vi "Cleanup.vi"(8 "error in (no error)":errorcluster, 11 "PanelArray in":refnum<class "PanelArray.lvclass">) -> (0 "error out":errorcluster)   [LabVIEW 2018, in "OOPanel.lvlib" / "PanelArray.lvclass"]
uses:
  PanelArray.lvclass
  PanelArray.lvclass/PanelArray.ctl
  Panel/Panel.lvclass
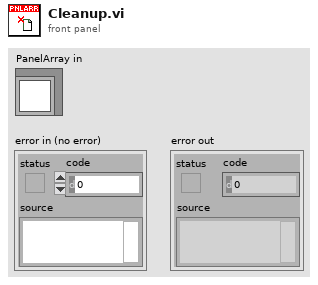
[diagram p1: front panel]
types:
  T1 = typedef "OOPanel.lvlib/PanelArray.lvclass/Ref Data.ctl" = cluster{"State":T2, "Refs":T3, "Events":T4, "Scrolling":T5, "Panels":T6}
  T2 = typedef "OOPanel.lvlib/PanelArray.lvclass/State.ctl" = cluster{"Defer Updates":bool, "Running":bool, "Dynamic Sizing":bool, "Borders":bool}
  T3 = typedef "OOPanel.lvlib/PanelArray.lvclass/Refs.ctl" = cluster{"SubPanels":refnum<vi>[], "Scrollbar":refnum<vi>, "Owning Panel":refnum<vi>}
  T4 = typedef "OOPanel.lvlib/PanelArray.lvclass/Events.ctl" = cluster{"Close":refnum<user-event>}
  T5 = typedef "OOPanel.lvlib/PanelArray.lvclass/Scrolling.ctl" = cluster{"Size":i32, "Max":i32, "Current":i32, "Top Index":i32, "Heights":i32[]}
  T6 = typedef "OOPanel.lvlib/PanelArray.lvclass/Panels.ctl" = cluster{"All":refnum<class "Panel.lvclass">[], "Visible":refnum<class "Panel.lvclass">[], "Blank":refnum<class "ArrayBlank.lvclass">}
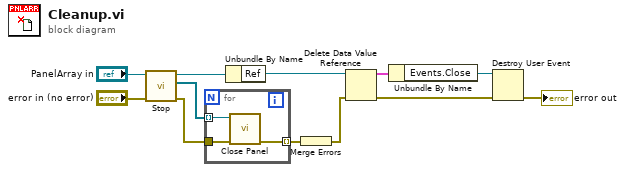
[diagram p0: block diagram]
diagram:
  n1 = call "Stop.vi"("error in (no error)"="error in (no error)", "PanelArray in"="PanelArray in") -> ("error out"=w4:errorcluster, "Remaining Panels"=w10:refnum<class "Panel.lvclass">[], "PanelArray out"=w9:refnum<class "PanelArray.lvclass">)  [unwired: 7 in]
  n2 = for {
    tunnel: w10 -> [w15] mode=indexing
    tunnel: [w14] -> w7 mode=indexing
    tunnel: w4 -> [w13]
    n3 = call "Close Panel.vi"("error in (no error)"=w13, "Panel in"=w15) -> ("error out"=w14:errorcluster)  [unwired: 8 in, 1 out]
  }
  n4 = Unbundle By Name(w9) -> ("Ref"=w8:refnum<data-value>)
  n5 = Merge Errors(w7) -> (w5:errorcluster)
  n6 = Delete Data Value Reference(data value reference=w8, error in=w5) -> (data value=w6:T1, error out=w2:errorcluster)
  n7 = Unbundle By Name(w6) -> ("Events.Close"=w3:refnum<user-event>)
  n8 = Destroy User Event(user event=w3, error in=w2) -> (error out=→"error out":errorcluster)
